vi "Get Target Temperature C.vi"(7 "Use Cached Data?":bool, 8 "Error In":errorcluster, 10 "Device Name":string, 11 "Nest Config":T1) -> (0 "Error Out":errorcluster, 1 "Target Temperature Low (C)":dbl, 2 "Target Temp (C)":dbl, 3 "Nest Config":T1, 5 "Target Temperature High (C)":dbl)   [LabVIEW 2013, in "LMH-Nest.lvlib"]
doc: "Get the target temperature of the specified Nest device."
uses:
  LMH-Nest.lvlib
  Private/Type Defs/Nest Config.ctl
  <vilib>/httpClient/ClientHandle.ctl
  Private/Type Defs/Session Data.ctl
  <vilib>/httpClient/LabVIEWHTTPClient.lvlib
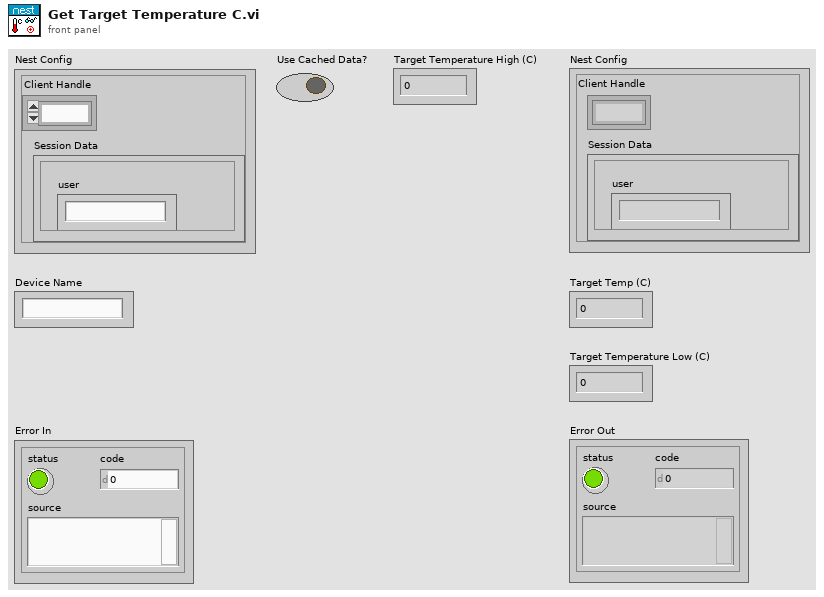
[diagram p1: front panel]
types:
  T1 = typedef "LMH-Nest.lvlib/Nest Config.ctl" = cluster{"Client Handle":T2, "Session Data":T3}
  T2 = typedef "LabVIEWHTTPClient.lvlib/ClientHandle.ctl" = refnum<k1>
  T3 = typedef "LMH-Nest.lvlib/Session Data.ctl" = cluster{"is_superuser":bool, "is_staff":bool, "urls":cluster{"transport_url":string, "rubyapi_url":string, "weather_url":string, "log_upload_url":string, "support_url":string}, "limits":cluster{"thermostats_per_structure":u32, "structures":u32, "thermostats":u32, "smoke_detectors":u32, "smoke_detectors_per_structure":u32}, "access_token":string, "userid":string, "expires_in":string, "email":string, "user":string, "language":string}
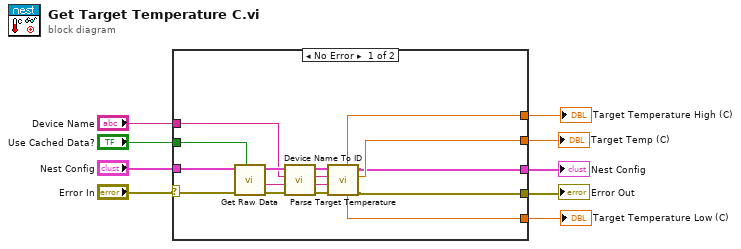
[diagram p0: block diagram]
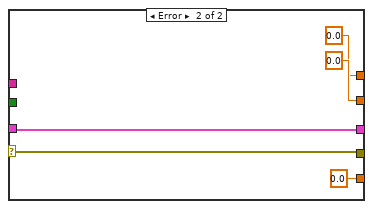
[diagram p2: hidden frame]
diagram:
  n1 = case shown="No Error" "Error In" {
    selector: "Error In" -> [w19 w30]
    tunnel: "Use Cached Data?" -> [w25 _]
    tunnel: "Nest Config" -> [w24 w29]
    tunnel: "Device Name" -> [w22 _]
    tunnel: [w14 w30] -> w6
    tunnel: [w12 w29] -> w5
    tunnel: [w13 0.0 ("Current Temp")] -> w4
    tunnel: [w11 0.0 ("Target Temperature Low (C)")] -> w2
    tunnel: [w10 0.0 ("Target Temperature High (C)")] -> w1
    frame No Error {
      n2 = call "Get Raw Data.vi"("Use Cached Data?"=w25, "Error In"=w19, "Nest Config"=w24) -> ("Error Out"=w21:errorcluster, "Data"=w20:string, "Nest Config"=w23:T1)  [unwired: 6 in]
      n3 = call "Device Name To ID.vi"("Error In"=w21, "Data"=w20, "Device Name"=w22, "Nest Config"=w23) -> ("Error Out"=w15:errorcluster, "Data"=w16:string, "Device ID"=w17:string, "Nest Config"=w18:T1)  [unwired: 4 in]
      n4 = call "Parse Target Temperature.vi"("Error In"=w15, "Data"=w16, "Device ID"=w17, "Nest Config"=w18) -> ("Error Out"=w14:errorcluster, "Target Temperature (C)"=w13:dbl, "Nest Config"=w12:T1, "Target Temperature Low (C)"=w11:dbl, "Target Temperature High (C)"=w10:dbl)  [unwired: 2 in, 1 out]
    }
    frame Error {
    }
  }
  "Error Out" <- w6
  "Nest Config" <- w5
  "Target Temp (C)" <- w4
  "Target Temperature High (C)" <- w1
  "Target Temperature Low (C)" <- w2
